vi "Configure Acquisition.vi"(4 "Reference Signal (0: Off)":i32(ring) items=["Off", "Out", "In"], 5 "Segment Count (2)":i32=2, 6 "Segment Index (1)":i32=1, 7 "Average Count (8)":dbl=8.0, 8 "error in (no error)":errorcluster, 9 "Acquisition Type (0: Normal)":i32(ring) items=["Normal", "Average", "High Resolution", "Peak"], 10 "Acquisition Format (0: Real-time)":i32(ring) items=["Real-time", "Segmented", "Equivalent-time", " Real-time (Max Update Rate)"], 11 "VISA resource name":refnum<visa-resource-name>) -> (0 "error out":errorcluster, 3 "VISA resource name out":refnum<visa-resource-name>)   [LabVIEW 2015, in "Agilent 2000 3000 X-Series.lvlib"]
doc: "Configure the acquisition settings."
uses:
  <instrlib>/Agilent 2000 3000 X-Series/Agilent 2000 3000 X-Series.lvlib
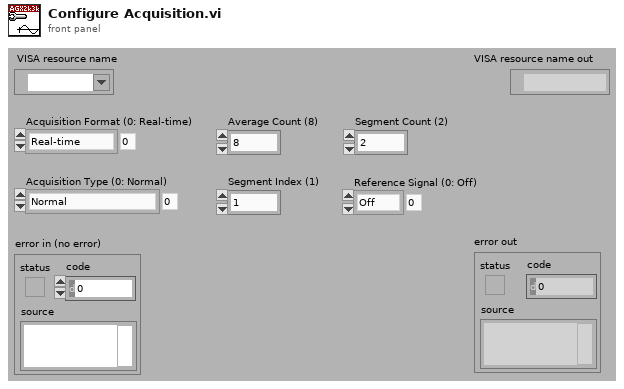
[diagram p1: front panel]
types:
  T1 = typedef "Agilent 2000 3000 X-Series.lvlib/Extended User Data.ctl" = cluster{"X-Series Mode":u16, "Acquisition Type (0: Normal)":i32}
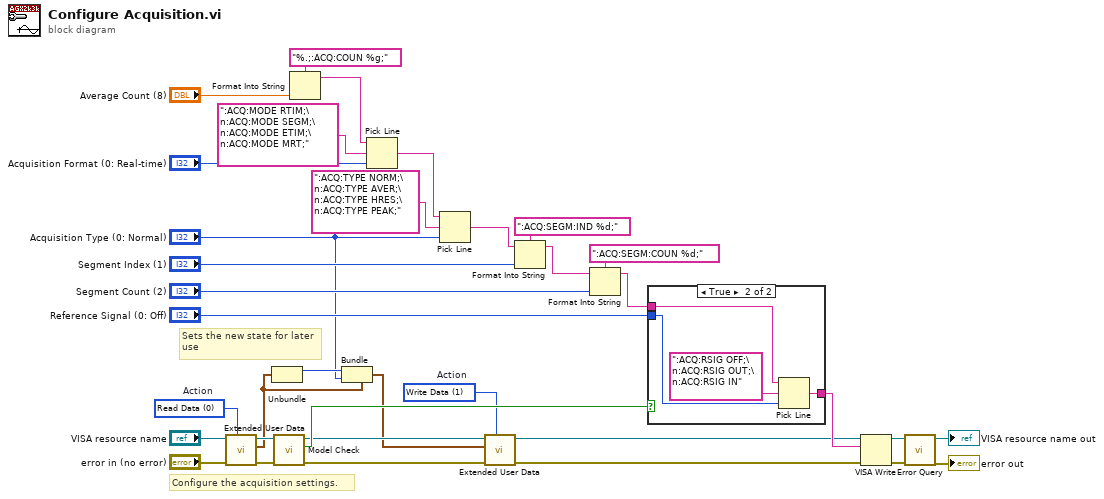
[diagram p0: block diagram]
diagram:
  w2 = 1 items=["Read Data", "Write Data", "Clear Data", "Clear ALL Data"]  # Action
  w6 = 0 items=["Read Data", "Write Data", "Clear Data", "Clear ALL Data"]  # Action
  # "Sets the new state for later\nuse"
  # "Configure the acquisition settings."
  n1 = call <instrlib>:"Extended User Data.vi"("Action (1: Write Data)"=w6, "error in (no error)"="error in (no error)", "VISA resource name in"="VISA resource name") -> ("error out"=w10:errorcluster, "User Data Out"=w1:T1, "VISA resource name out"=w9:refnum<visa-resource-name>)  [unwired: 6 in]
  n2 = Unbundle(w1) -> ("X-Series Mode"=w5:u16)  [unwired: 1 out]
  n3 = call <instrlib>:"Model Check.vi"("error in (no error)"=w10, "VISA resource name"=w9) -> ("error out"=w14:errorcluster, "Not 2000 or 3000 Series"=w15:bool, "VISA resource name out"=w13:refnum<visa-resource-name>)  [unwired: 7 out]
  n4 = Format Into String(format string="%.;:ACQ:COUN %g;", "Average Count (8)") -> (resulting string=w31:string)  [unwired: 2 in, 1 out]
  n5 = Bundle(cluster=w1, "X-Series Mode"=w5, "Acquisition Type (0: Normal)"="Acquisition Type (0: Normal)") -> (w3:T1)
  n6 = Pick Line(string ("")=w31, multi-line string=":ACQ:MODE RTIM;\n:ACQ:MODE SEGM;\n:ACQ:MODE ETIM;\n:ACQ:MODE MRT;", line index="Acquisition Format (0: Real-time)") -> (output string=w29:string)
  n7 = Pick Line(string ("")=w29, multi-line string=":ACQ:TYPE NORM;\n:ACQ:TYPE AVER;\n:ACQ:TYPE HRES;\n:ACQ:TYPE PEAK;", line index="Acquisition Type (0: Normal)") -> (output string=w28:string)
  n8 = call <instrlib>:"Extended User Data.vi"("Action (1: Write Data)"=w2, "error in (no error)"=w14, "User Data In"=w3, "VISA resource name in"=w13) -> ("error out"=w11:errorcluster, "VISA resource name out"=w12:refnum<visa-resource-name>)  [unwired: 5 in, 1 out]
  n9 = Format Into String(format string=":ACQ:SEGM:IND %d;", initial string=w28, "Segment Index (1)") -> (resulting string=w25:string)  [unwired: 1 in, 1 out]
  n10 = Format Into String(format string=":ACQ:SEGM:COUN %d;", initial string=w25, "Segment Count (2)") -> (resulting string=w18:string)  [unwired: 1 in, 1 out]
  n11 = case shown="True" w15 {
    tunnel: w18 -> [w36 w39]
    tunnel: [w36 w38] -> w16
    tunnel: "Reference Signal (0: Off)" -> [_ w37]
    frame False {
    }
    frame True {
      n12 = Pick Line(string ("")=w39, multi-line string=":ACQ:RSIG OFF;\n:ACQ:RSIG OUT;\n:ACQ:RSIG IN", line index=w37) -> (output string=w38:string)
    }
  }
  n13 = VISA Write(VISA resource name=w12, write buffer=w16, error in (no error)=w11) -> (VISA resource name out=w22:refnum<visa-resource-name>, error out=w21:errorcluster)  [unwired: 1 out]
  n14 = call <instrlib>:"Error Query.vi"("error in (no error)"=w21, "VISA resource name"=w22) -> ("error out"=→"error out":errorcluster, "VISA resource name out"=→"VISA resource name out":refnum<visa-resource-name>)  [unwired: 8 out]
